vi "Gif.Main.vi"(0 "file path":path, 9 "bgcolor":u32(colorbox)=16777226, 11 "error in (no error)":errorcluster, 12 "image index":i32) -> (6 "time":u32[](array[numeric]), 8 "images out":picture[](array[picture]), 13 "image data":T1, 14 "image size":cluster{"Width":u32, "Height":u32}, 15 "error out":errorcluster)   [LabVIEW 2019]
doc: "This VI reads all images from a gif file.\nCurrently it can only read from version 89a.\nInterlaced images are not taken into account.\n\nThe outputs are an array of all delay times, an array of all images, the image size and an error cluster.\n\nVersion 01.01\nMike Schröder"
uses:
  <vilib>/picture/picture.llb/imagedata.ctl
panel:
  out "color table":u32[](array[colorbox])
  out "Version":string
  out "Signature":string
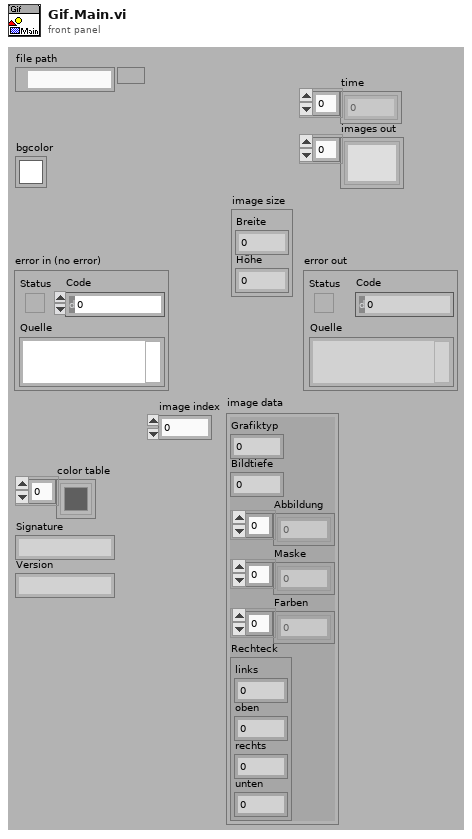
[diagram p1: front panel]
types:
  T1 = typedef "imagedata.ctl" = cluster{"image type":i32, "image depth":i32, "image":u8[], "mask":u8[], "colors":u32[], "Rectangle":cluster{"left":i16, "top":i16, "right":i16, "bottom":i16}}
  T2 = enum16{"deny read/write", "deny write-only", "deny none"}
  T3 = enum16{"read/write", "read-only", "write-only", "write-only (truncate)"}
  T4 = typedef "Gif.LogicalScreenDescriptior.ctl" = cluster{"Logical Screen Width":u16, "Logical Screen Height":u16, "Global Color Table Flag":u8, "Color Resolution":u8, "Sort Flag":u8, "Size of Global Color Table":u8, "Background Color Index":u8, "Pixel Aspect Ratio":u8}
  T5 = typedef "Gif.GraphicControlExtension.ctl" = cluster{"Reserved":u8, "Disposal Method":u8, "User Input Flag":u8, "Transparent Color Flag":u8, "Delay Time":u16, "Transparent Color Index":u8}
  T6 = typedef "Gif.ImageDescriptor.ctl" = cluster{"Image Left Position":u16, "Image Top Position":u16, "Image Width":u16, "Image Height":u16, "Local Color Table Flag":u8, "Interlace Flag":u8, "Sort Flag":u8, "Reserved":u8, "Size Of Local Color Table":u8}
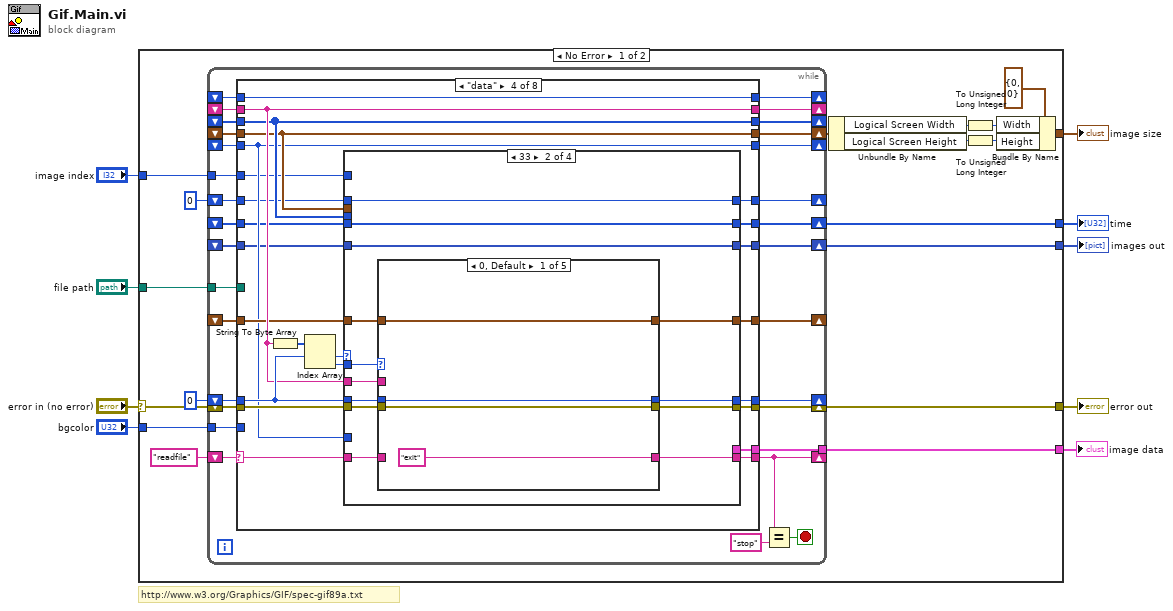
[diagram p0: block diagram]
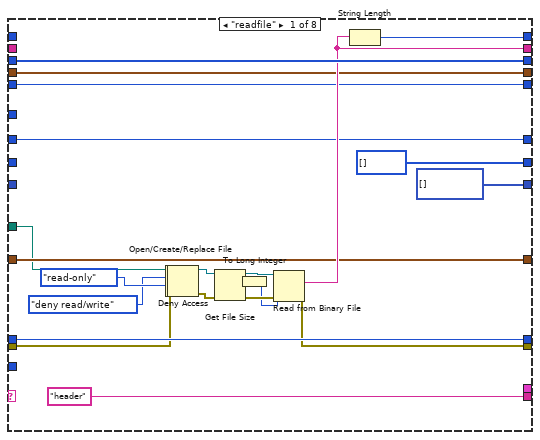
[diagram p2: hidden frame]
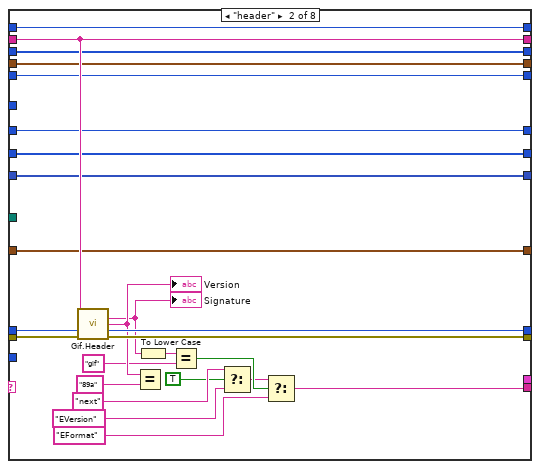
[diagram p3: hidden frame]
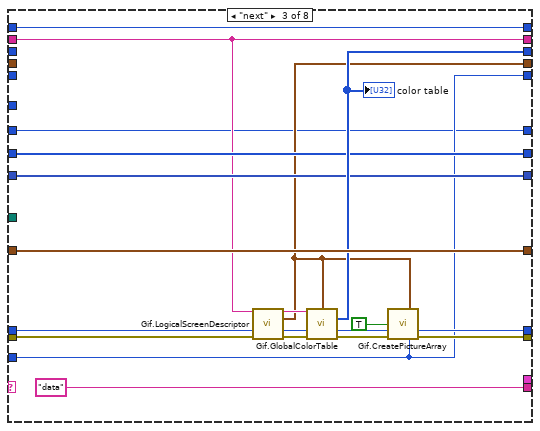
[diagram p4: hidden frame]
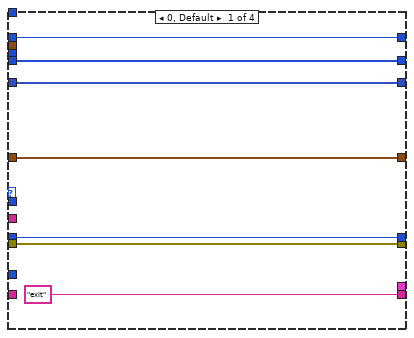
[diagram p5: hidden frame]
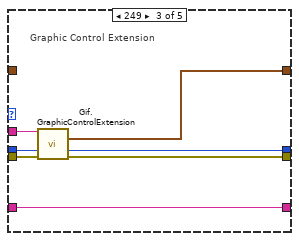
[diagram p7: hidden frame]
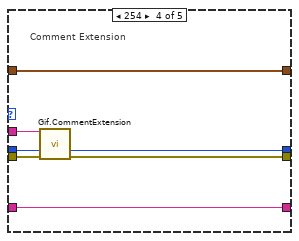
[diagram p8: hidden frame]
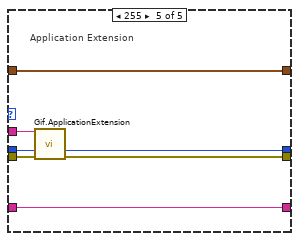
[diagram p9: hidden frame]
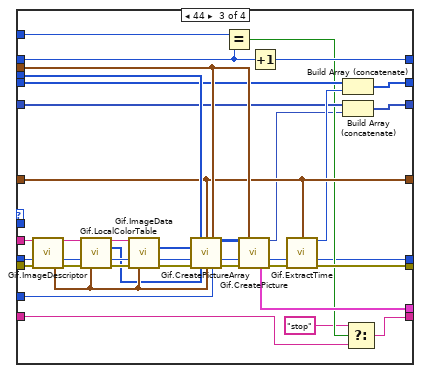
[diagram p10: hidden frame]
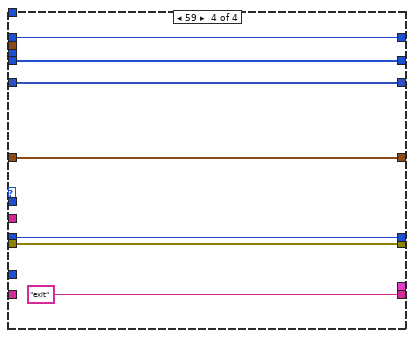
[diagram p11: hidden frame]
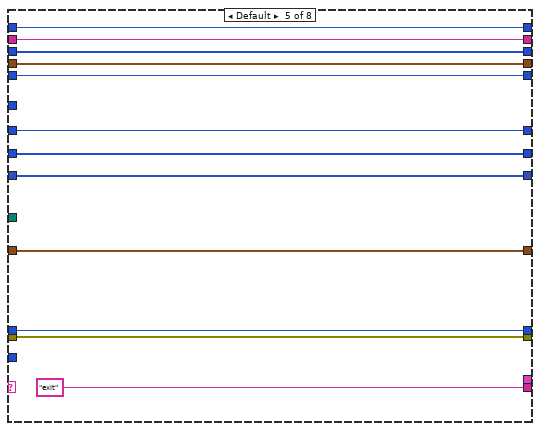
[diagram p12: hidden frame]
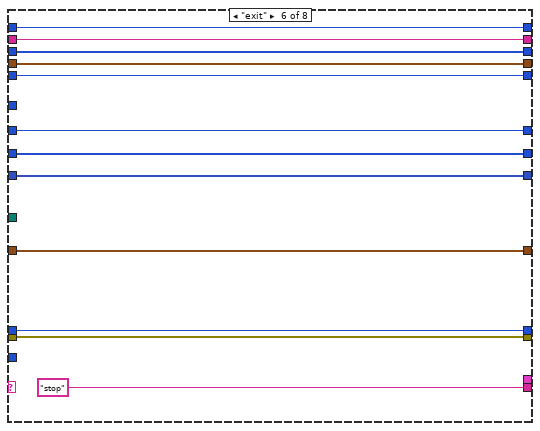
[diagram p13: hidden frame]
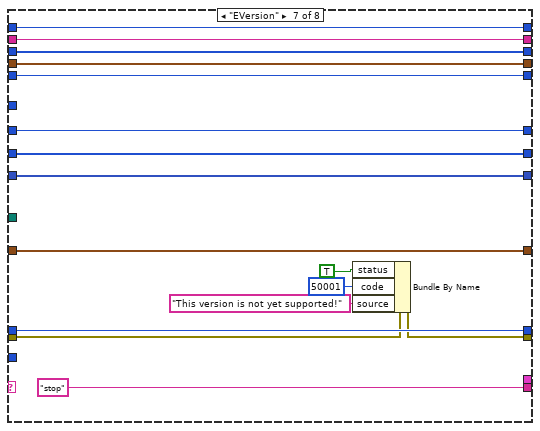
[diagram p14: hidden frame]
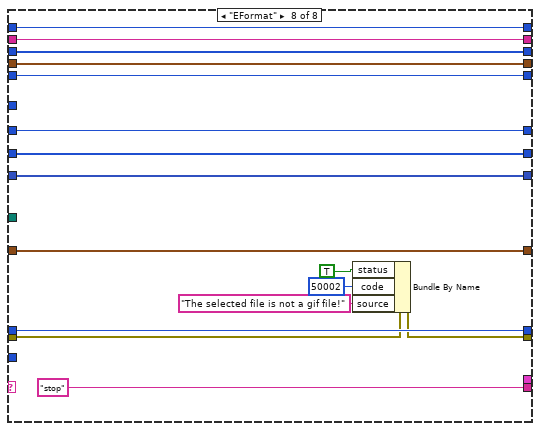
[diagram p15: hidden frame]
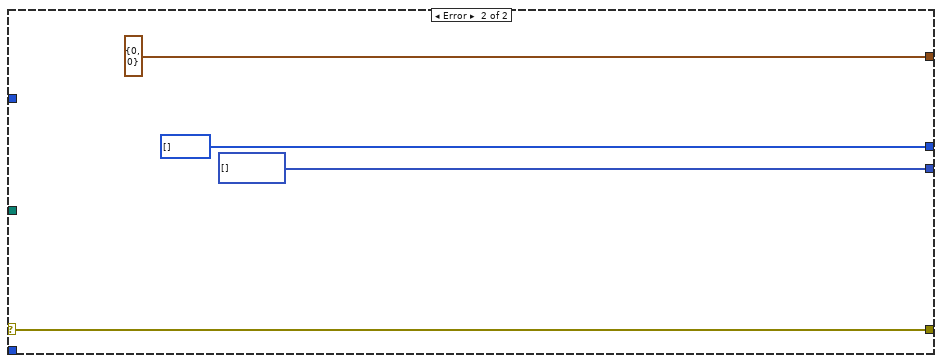
[diagram p16: hidden frame]
diagram:
  # "http://www.w3.org/Graphics/GIF/spec-gif89a.txt"
  n1 = case shown="No Error" "error in (no error)" {
    selector: "error in (no error)" -> [w13 w305]
    tunnel: [w25 u32[] []] -> w9
    tunnel: [w24 picture[] []] -> w1
    tunnel: "bgcolor" -> [w22 _]
    tunnel: "file path" -> [w21 _]
    tunnel: [w20 w305] -> w6
    tunnel: [w14 cluster{"Width":u32, "Height":u32} {"Width"=0, "Height"=0} ("Größe des Darstellungsbereichs")] -> w5
    tunnel: "image index" -> [w11 _]
    tunnel: [w10 _] -> w2
    frame No Error {
      n2 = while {
        shift-right: [w48] -> _
        shift-left: "readfile" -> [w57]
        shift-right: [w56] -> _
        shift-left: _ -> [w54]
        shift-right: [w55] -> _
        shift-left: _ -> [w53]
        shift-right: [w51] -> w20
        shift-left: w13 -> [w52]
        shift-right: [w49] -> _
        shift-left: 0 ("offset (0)") -> [w50]
        shift-right: [w45] -> _
        shift-left: _ -> [w44]
        shift-right: [w43] -> _
        shift-left: _ -> [w42]
        shift-right: [w41] -> w23
        shift-left: _ -> [w40]
        shift-right: [w39] -> _
        shift-left: _ -> [w38]
        shift-right: [w36] -> w25
        shift-left: _ -> [w37]
        shift-right: [w34] -> w24
        shift-left: _ -> [w35]
        tunnel: w22 -> [w33]
        tunnel: w21 -> [w32]
        shift-right: [w29] -> _
        shift-left: 0 ("offset (0)") -> [w30]
        tunnel: w11 -> [w28]
        tunnel: [w31] -> w10
        stop <- w46 stop-if-true
        n3 = case shown="\"data\"" w57 {
          selector: w57 -> [_ _ _ w141 _ _ _ _]
          tunnel: [w81 w106 w126 w150 w257 w269 w285 w301] -> w56
          tunnel: [w77 w104 w110 w140 w256 w268 w284 w300] -> w55
          tunnel: w54 -> [_ w106 w126 w150 w257 w269 w285 w301]
          tunnel: w53 -> [_ w104 w110 w140 w256 w268 w284 w300]
          tunnel: ["header" w85 "data" w142 "exit" "stop" "stop" "stop"] -> w48
          tunnel: w52 -> [w69 w105 w109 w145 w254 w266 w275 w291]
          tunnel: [w68 w99 w113 w144 w254 w266 w274 w290] -> w51
          tunnel: w50 -> [w79 w103 w108 w146 w253 w265 w282 w298]
          tunnel: [w79 w98 w115 w143 w253 w265 w282 w298] -> w49
          tunnel: [w78 w97 w120 w139 w252 w264 w281 w297] -> w45
          tunnel: w44 -> [w78 w97 _ w139 w252 w264 w281 w297]
          tunnel: [w74 w102 w124 w138 w251 w263 w280 w296] -> w43
          tunnel: w42 -> [w74 w102 w124 w137 w251 w263 w280 w296]
          tunnel: [w73 w96 w112 w136 w250 w262 w279 w295] -> w41
          tunnel: w40 -> [w73 w96 _ w136 w250 w262 w279 w295]
          tunnel: [w72 w95 w111 w135 w249 w261 w278 w294] -> w39
          tunnel: w38 -> [w72 w95 _ w135 w249 w261 w278 w294]
          tunnel: w37 -> [_ w101 w119 w134 w248 w260 w277 w293]
          tunnel: [u32[] [] w101 w119 w133 w248 w260 w277 w293] -> w36
          tunnel: w35 -> [_ w100 w118 w132 w247 w259 w276 w292]
          tunnel: [picture[] [] w100 w118 w131 w247 w259 w276 w292] -> w34
          tunnel: w33 -> [_ _ w111 _ _ _ _ _]
          tunnel: w32 -> [w70 _ _ _ _ _ _ _]
          tunnel: [_ _ _ w130 _ _ _ _] -> w31
          tunnel: w30 -> [w67 w82 w107 w129 w246 w258 w270 w286]
          tunnel: [w67 w82 w107 w128 w246 w258 w270 w286] -> w29
          tunnel: w28 -> [_ _ _ w127 _ _ _ _]
          frame "readfile" {
            n4 = Open/Create/Replace File(file path (use dialog)=w70, error in=w69, access (0:read/write)=T3."read-only" ("open mode (0)")) -> (refnum out=w58:refnum<file>, error out=w59:errorcluster)  [unwired: 3 in, 1 out]
            n5 = Deny Access(4:w59, 6:T2."deny read/write" ("deny mode (2)"), 7:w58) -> (0:w64:errorcluster, 3:w65:refnum<file>)
            n6 = Get File Size(file=w65, error in=w64) -> (refnum out=w75:refnum<file>, size (in bytes)=w60:i64, 0:w76:errorcluster)
            n7 = To Long Integer(number=w60) -> (32bit integer=w63:i32)
            n8 = Read from Binary File(8:w76, 10:w63, 11:w75) -> (0:w68:errorcluster, 2:w77:string)  [unwired: 3 in, 2 out]
            n9 = String Length(string=w77) -> (length=w81:i32)
          }
          frame "header" {
            n10 = call "Gif.Header.vi"("data"=w104, "offset"=w103, "error in (no error)"=w105) -> ("Signature"=w90:string, "Version"=w94:string, "offset out"=w98:i32, "error out"=w99:errorcluster)  [unwired: 1 in, 8 out]
            "Signature" <- w90
            "Version" <- w94
            n11 = Equal?(x=w94, y="89a") -> ()  [unwired: 1 out]
            n12 = To Lower Case(string=w90) -> (all lower case string=w89:string)
            n13 = Equal?(x=w89, y="gif") -> (x = y?=w87:bool)
            n14 = Select(t="next", s=TRUE, f="EVersion") -> (s? t:f=w86:string)
            n15 = Select(t=w86, s=w87, f="EFormat") -> (s? t:f=w85:string)
          }
          frame "next" {
            n16 = call "Gif.LogicalScreenDescriptor.vi"("data"=w110, "offset"=w108, "error in (no error)"=w109) -> ("data out"=w121:string, "Logical Screen Descriptor"=w112:T4, "offset out"=w122:i32, "error out"=w123:errorcluster)  [unwired: 9 out]
            n17 = call "Gif.GlobalColorTable.vi"("data"=w121, "Logical Screen Descriptor"=w112, "offset"=w122, "error in (no error)"=w123) -> ("global color table"=w120:u32[], "offset out"=w116:i32, "error out"=w114:errorcluster)  [unwired: 1 in, 8 out]
            "color table" <- w120
            n18 = call "Gif.CreatePictureArray.vi"("Logical Screen Description"=w112, "init"=TRUE, "offset"=w116, "error in (no error)"=w114, "bgcolor"=w111) -> ("offset out"=w115:i32, "error out"=w113:errorcluster)  [unwired: 5 in, 4 out]
          }
          frame "data" {
            n19 = String To Byte Array(string=w140) -> (unsigned byte array=w149:u8[])
            n20 = Index Array(array=w149, index #1=w146) -> (element #1=w148:u8, element #2=w147:u8)  [unwired: 1 in]
            n21 = case shown="33" w148 {
              tunnel: w147 -> [_ w170 _ _]
              tunnel: w146 -> [w156 w166 w237 w244]
              tunnel: w145 -> [w157 w165 w238 w243]
              tunnel: [w157 w164 w212 w243] -> w144
              tunnel: [w156 w167 w202 w244] -> w143
              tunnel: ["exit" w169 w204 "exit"] -> w142
              tunnel: w141 -> [_ w168 w206 _]
              tunnel: w140 -> [_ w163 w236 _]
              tunnel: w139 -> [_ _ w222 _]
              tunnel: [w154 w162 w220 w242] -> w138
              tunnel: w137 -> [w154 w161 w220 w242]
              tunnel: w136 -> [_ _ w221 _]
              tunnel: w135 -> [_ _ w219 _]
              tunnel: w134 -> [w153 w160 w218 w241]
              tunnel: [w153 w160 w216 w241] -> w133
              tunnel: w132 -> [w152 w159 w215 w240]
              tunnel: [w152 w159 w214 w240] -> w131
              tunnel: [_ _ w210 _] -> w130
              tunnel: w129 -> [w151 w158 w200 w239]
              tunnel: [w151 w158 w208 w239] -> w128
              tunnel: w127 -> [_ _ w209 _]
              frame 0, Default {
              }
              frame 33 {
                n22 = case shown="0, Default" w170 {
                  tunnel: ["exit" w178 w185 w192 w199] -> w169
                  tunnel: w168 -> [_ w178 w185 w192 w199]
                  tunnel: [w173 w177 w181 w189 w197] -> w167
                  tunnel: w166 -> [w173 w177 w183 w190 w198]
                  tunnel: w165 -> [w172 w176 w184 w191 w196]
                  tunnel: [w172 w176 w182 w188 w195] -> w164
                  tunnel: w163 -> [_ _ w180 w187 w194]
                  tunnel: [w171 w175 w179 w186 w193] -> w162
                  tunnel: w161 -> [w171 w175 _ w186 w193]
                  frame 0, Default {
                  }
                  frame 1 {
                  }
                  frame 249 {
                    # "Graphic Control Extension"
                    n23 = call "Gif.GraphicControlExtension.vi"("data"=w180, "offset"=w183, "error in (no error)"=w184) -> ("GraphicControlExtension"=w179:T5, "offset out"=w181:i32, "error out"=w182:errorcluster)  [unwired: 10 out]
                  }
                  frame 254 {
                    # "Comment Extension"
                    n24 = call "Gif.CommentExtension.vi"("data"=w187, "offset"=w190, "error in (no error)"=w191) -> ("offset out"=w189:i32, "error out"=w188:errorcluster)  [unwired: 11 out]
                  }
                  frame 255 {
                    # "Application Extension"
                    n25 = call "Gif.ApplicationExtension.vi"("data"=w194, "offset"=w198, "error in (no error)"=w196) -> ("offset out"=w197:i32, "error out"=w195:errorcluster)  [unwired: 11 out]
                  }
                }
              }
              frame 44 {
                n26 = call "Gif.ImageDescriptor.vi"("data"=w236, "offset"=w237, "error in (no error)"=w238) -> ("data out"=w233:string, "offset out"=w234:i32, "ImageDescriptor"=w224:T6, "error out"=w235:errorcluster)  [unwired: 9 out]
                n27 = call "Gif.LocalColorTable.vi"("data"=w233, "offset"=w234, "error in (no error)"=w235, "ImageDescriptor"=w224) -> ("data out"=w230:string, "local color table"=w223:u32[], "offset out"=w231:i32, "error out"=w232:errorcluster)  [unwired: 5 in, 3 out]
                n28 = call "Gif.ImageData.vi"("data"=w230, "offset"=w231, "error in (no error)"=w232, "ImageDescriptor"=w224) -> ("Index Array"=w228:i32[], "offset out"=w203:i32, "error out"=w229:errorcluster)  [unwired: 1 in, 8 out]
                n29 = call "Gif.CreatePictureArray.vi"("gloal color table"=w222, "GraphicControlExtension"=w220, "Logical Screen Description"=w221, "Index Array"=w228, "offset"=w203, "error in (no error)"=w229, "local color table"=w223, "ImageDescriptor"=w224, "bgcolor"=w219) -> ("image out"=w225:u32[][], "offset out"=w226:i32, "error out"=w227:errorcluster)  [unwired: 1 in, 3 out]
                n30 = Equal?(x=w209, y=w200) -> (x = y?=w207:bool)
                n31 = call "Gif.CreatePicture.vi"("image in"=w225, "Logical Screen Description"=w221, "offset"=w226, "error in (no error)"=w227) -> ("image out"=w201:picture, "offset out"=w211:i32, "graphic data"=w210:T1, "error out"=w213:errorcluster)  [unwired: 8 out]
                n32 = Increment(x=w200) -> (x+1=w208:i32)
                n33 = call "Gif.ExtractTime.vi"("GraphicControlExtension"=w220, "offset"=w211, "error in (no error)"=w213) -> ("time"=w217:u32, "offset out"=w202:i32, "error out"=w212:errorcluster)  [unwired: 10 out]
                n34 = Build Array (concatenate)(w218, w217) -> (w216:u32[])
                n35 = Build Array (concatenate)(w215, w201) -> (w214:picture[])
                n36 = Select(t="stop", s=w207, f=w206) -> (s? t:f=w204:string)
              }
              frame 59 {
              }
            }
          }
          frame Default {
          }
          frame "exit" {
          }
          frame "EVersion" {
            n37 = Bundle By Name(cluster=w275, "status"=TRUE, "code"=50001, "source"="This version is not yet supported!") -> (w274:errorcluster)
          }
          frame "EFormat" {
            n38 = Bundle By Name(cluster=w291, "status"=TRUE, "code"=50002, "source"="The selected file is not a gif file!") -> (w290:errorcluster)
          }
        }
        n39 = Equal?(x=w48, y="stop") -> (x = y?=w46:bool)
      }
      n40 = Unbundle By Name(w23) -> ("Logical Screen Width"=w17:u16, "Logical Screen Height"=w16:u16)
      n41 = To Unsigned Long Integer(number=w17) -> (unsigned 32bit integer=w18:u32)
      n42 = To Unsigned Long Integer(number=w16) -> (unsigned 32bit integer=w19:u32)
      n43 = Bundle By Name(cluster=cluster{"Width":u32, "Height":u32} {"Width"=0, "Height"=0} ("Größe des Darstellungsbereichs"), "Width"=w18, "Height"=w19) -> (w14:cluster{"Width":u32, "Height":u32})
    }
    frame Error {
    }
  }
  "time" <- w9
  "error out" <- w6
  "image size" <- w5
  "image data" <- w2
  "images out" <- w1
